vi "add_light.vi"(9 "Lights":T1, 10 "Lighting Properties":T2, 11 "Scene:New Object":refnum<vi>) -> (3 "Scene:New Object 2":refnum<vi>)   [LabVIEW 2020, in "3DPC_SurfacePlot.xctl"]
uses:
  <vilib>/Native 3D Graph/xcontrol/3DPC_SurfacePlot.xctl
  <vilib>/Native 3D Graph/typedefs/prop_lighting.ctl
  <vilib>/Native 3D Graph/typedefs/prop_lights.ctl
  <vilib>/picture/3D Picture Control/NI_3D Picture Control.lvlib
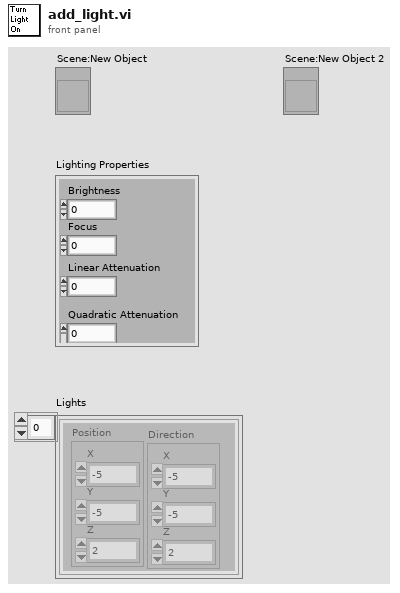
[diagram p1: front panel]
types:
  T1 = typedef "3DPC_SurfacePlot.xctl/prop_lights.ctl" = cluster{"Position":cluster{"X":sgl, "Y":sgl, "Z":sgl}, "Direction":cluster{"X":sgl, "Y":sgl, "Z":sgl}}[]
  T2 = typedef "3DPC_SurfacePlot.xctl/prop_lighting.ctl" = cluster{"Brightness":i32, "Focus":dbl, "Linear Attenuation":dbl, "Quadratic Attenuation":dbl}
  T3 = typedef "LVAttenuationTypeDef.ctl" = cluster{"Constant":sgl, "Linear":sgl, "Quadratic":sgl}
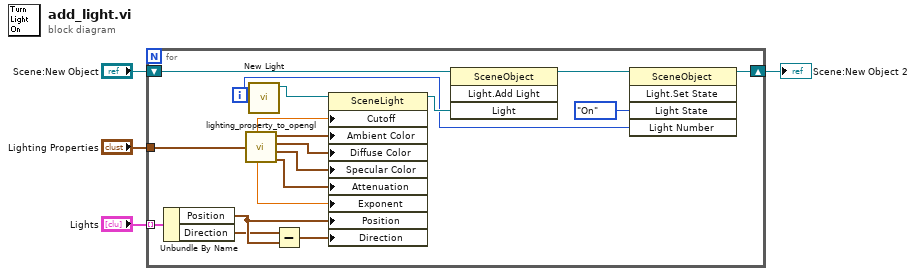
[diagram p0: block diagram]
diagram:
  n1 = for {
    tunnel: "Lighting Properties" -> [w20]
    tunnel: "Lights" -> [w15] mode=indexing
    shift-right: [w9] -> w1
    shift-left: "Scene:New Object" -> [w22]
    i -> [w7]
    n2 = Unbundle By Name(w15) -> ("Position"=w14:cluster{"X":sgl, "Y":sgl, "Z":sgl}, "Direction"=w13:cluster{"X":sgl, "Y":sgl, "Z":sgl})
    n3 = call <vilib>:"lighting_property_to_opengl.vi"("Lighting Properties"=w20) -> ("Cutoff"=w19:dbl, "Exponent"=w16:dbl, "Ambient Color"=w18:cluster{"R":sgl, "G":sgl, "B":sgl, "A":sgl}, "Diffuse Color"=w5:cluster{"R":sgl, "G":sgl, "B":sgl, "A":sgl}, "Specular Color"=w6:cluster{"R":sgl, "G":sgl, "B":sgl, "A":sgl}, "Attenuation"=w17:T3)  [unwired: 2 out]
    n4 = call <vilib>:"New Light.vi"("Light Number"=w7) -> ("New Light Refnum"=w21:refnum<vi>)  [unwired: 2 in, 8 out]
    n5 = Subtract(x=w13, y=w14) -> (x-y=w12:cluster{"X":sgl, "Y":sgl, "Z":sgl})
    n6 = property class="SceneLight"(reference=w21, "Cutoff"=w19, "Ambient Color"=w18, "Diffuse Color"=w5, "Specular Color"=w6, "Attenuation"=w17, "Exponent"=w16, "Position"=w14, "Direction"=w12) -> (reference out=w11:refnum<vi>)  [unwired: 1 in, 1 out]
    n7 = invoke class="SceneObject" method="Light.Add Light"(reference=w22, "Light"=w11) -> (reference out=w10:refnum<vi>)  [unwired: 2 in, 3 out]
    n8 = invoke class="SceneObject" method="Light.Set State"(reference=w10, "Light State"=enum16{"Inherit Value", "Off", "On"}."On", "Light Number"=w7) -> (reference out=w9:refnum<vi>)  [unwired: 2 in, 4 out]
  }
  "Scene:New Object 2" <- w1
